vi "Add Node.vi"(6 "Display Name":string, 8 "error in (no error)":errorcluster, 9 "UID":string, 10 "Parent":string, 11 "Base Tree in":refnum<class "Base Tree.lvclass">) -> (0 "error out":errorcluster, 3 "Base Tree out":refnum<class "Base Tree.lvclass">)   [LabVIEW 2017, in "opcua.lvlib" / "Browser Core.lvlib" / "Base Tree.lvclass"]
doc: "Create node with given UID and Add it as a child to the given Parent node. If the Parent input is empty, the node will be treated as a child of the Root Node."
uses:
  Base Tree.lvclass
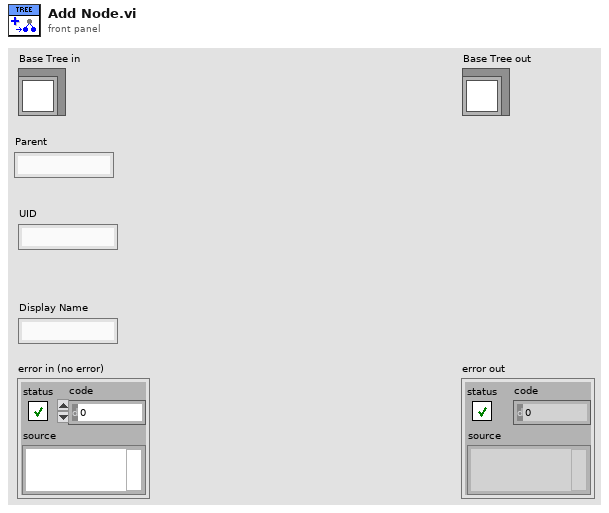
[diagram p1: front panel]
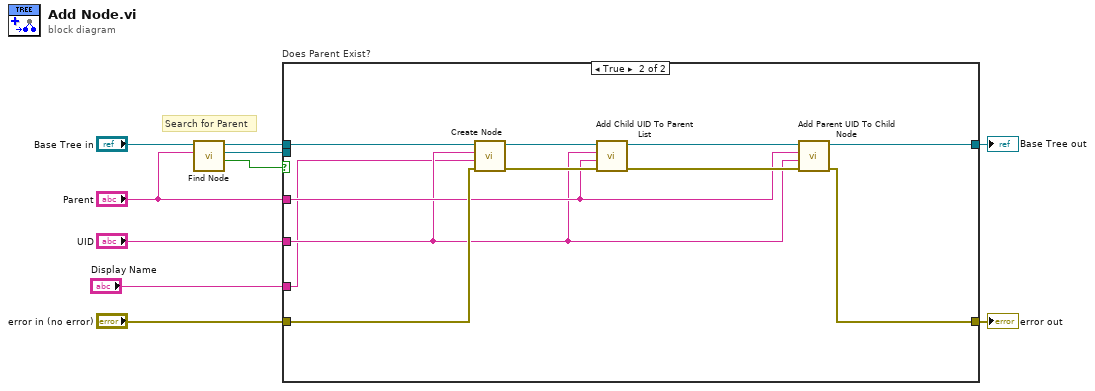
[diagram p0: block diagram]
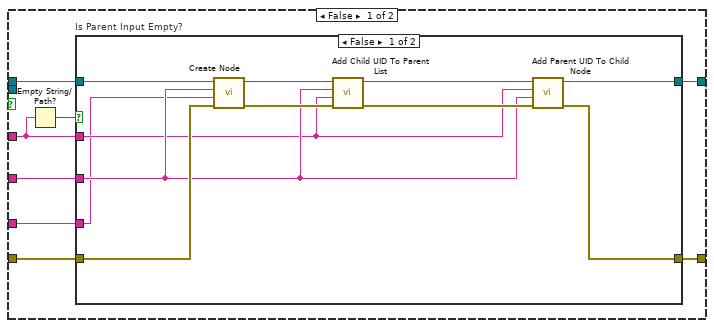
[diagram p2: hidden frame]
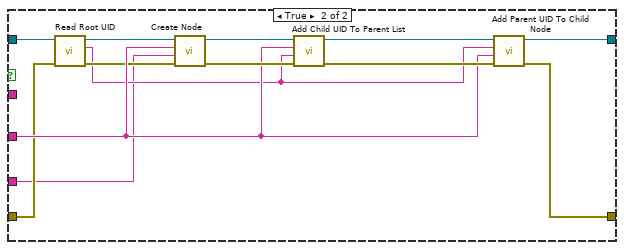
[diagram p3: hidden frame]
diagram:
  # "Search for Parent"
  n1 = call-dynamic "Find Node.vi"("UID"="Parent", "Base Tree in"="Base Tree in") -> ("Found?"=w5:bool, "Node"=w4:refnum<class "Generic Node.lvclass">, "Base Tree out"=w6:refnum<class "Base Tree.lvclass">)  [unwired: 6 in, 1 out]
  n2 = case "Does Parent Exist?" shown="True" w5 {
    tunnel: "error in (no error)" -> [w14 w51]
    tunnel: [w18 w46] -> w8
    tunnel: [w16 w48] -> w7
    tunnel: w6 -> [w17 w53]
    tunnel: w4 -> [_ _]
    tunnel: "UID" -> [w13 w44]
    tunnel: "Parent" -> [w12 w45]
    tunnel: "Display Name" -> [w11 w43]
    frame False {
      n3 = Empty String/Path?(string/path=w12) -> (empty?=w15:bool)
      n4 = case "Is Parent Input Empty?" shown="False" w15 {
        tunnel: [w22 w37] -> w18
        tunnel: w17 -> [w29 w35]
        tunnel: [w24 w39] -> w16
        tunnel: w14 -> [w28 w33]
        tunnel: w13 -> [w21 w36]
        tunnel: w12 -> [w20 _]
        tunnel: w11 -> [w19 w30]
        frame False {
          n5 = call "Create Node.vi"("error in (no error)"=w28, "Display Name"=w19, "UID"=w21, "Base Tree in"=w29) -> ("error out"=w26:errorcluster, "Base Tree out"=w27:refnum<class "Base Tree.lvclass">)  [unwired: 6 in]
          n6 = call "Add Child UID To Parent List.vi"("Base Tree in"=w27, "UID"=w21, "ParentUID"=w20, "error in (no error)"=w26) -> ("Base Tree out"=w25:refnum<class "Base Tree.lvclass">, "error out"=w23:errorcluster)  [unwired: 5 in]
          n7 = call "Add Parent UID To Child Node.vi"("error in (no error)"=w23, "Child UID"=w21, "Parent UID"=w20, "Base Tree in"=w25) -> ("error out"=w22:errorcluster, "Base Tree out"=w24:refnum<class "Base Tree.lvclass">)  [unwired: 5 in, 1 out]
        }
        frame True {
          n8 = call "Read Root UID.vi"("error in (no error)"=w33, "Base Tree in"=w35) -> ("error out"=w32:errorcluster, "Root UID"=w31:string, "Base Tree out"=w34:refnum<class "Base Tree.lvclass">)  [unwired: 7 in]
          n9 = call "Create Node.vi"("error in (no error)"=w32, "Display Name"=w30, "UID"=w36, "Base Tree in"=w34) -> ("error out"=w41:errorcluster, "Base Tree out"=w42:refnum<class "Base Tree.lvclass">)  [unwired: 6 in]
          n10 = call "Add Child UID To Parent List.vi"("Base Tree in"=w42, "UID"=w36, "ParentUID"=w31, "error in (no error)"=w41) -> ("Base Tree out"=w40:refnum<class "Base Tree.lvclass">, "error out"=w38:errorcluster)  [unwired: 5 in]
          n11 = call "Add Parent UID To Child Node.vi"("error in (no error)"=w38, "Child UID"=w36, "Parent UID"=w31, "Base Tree in"=w40) -> ("error out"=w37:errorcluster, "Base Tree out"=w39:refnum<class "Base Tree.lvclass">)  [unwired: 5 in, 1 out]
        }
      }
    }
    frame True {
      n12 = call "Create Node.vi"("error in (no error)"=w51, "Display Name"=w43, "UID"=w44, "Base Tree in"=w53) -> ("error out"=w50:errorcluster, "Base Tree out"=w52:refnum<class "Base Tree.lvclass">)  [unwired: 6 in]
      n13 = call "Add Child UID To Parent List.vi"("Base Tree in"=w52, "UID"=w44, "ParentUID"=w45, "error in (no error)"=w50) -> ("Base Tree out"=w49:refnum<class "Base Tree.lvclass">, "error out"=w47:errorcluster)  [unwired: 5 in]
      n14 = call "Add Parent UID To Child Node.vi"("error in (no error)"=w47, "Child UID"=w44, "Parent UID"=w45, "Base Tree in"=w49) -> ("error out"=w46:errorcluster, "Base Tree out"=w48:refnum<class "Base Tree.lvclass">)  [unwired: 5 in, 1 out]
    }
  }
  "error out" <- w8
  "Base Tree out" <- w7
